vi "DM API.vi"(4 "response timeout(500)":i32=500, 6 "response":bool, 8 "error in (no error)":errorcluster, 10 "parameters":string, 11 "message":string) -> (0 "error out":errorcluster, 1 "data":variant, 2 "response":string, 3 "status":string)   [LabVIEW 2019, in "DataManagment.lvlib"]
uses:
  DataManagment.lvlib
  Intertarget communication/Command + data + response cluster.ctl
  Intertarget communication/Status + response + data cluster.ctl
  DM GV.vi
  Intertarget communication/CommandResponse communication.lvlib
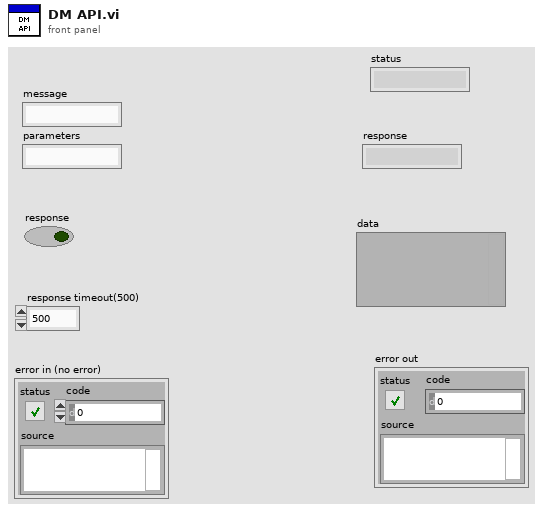
[diagram p1: front panel]
types:
  T1 = typedef "CommandResponse communication.lvlib/Status + response + data cluster.ctl" = cluster{"message":string, "response":string, "data":variant}
  T2 = typedef "CommandResponse communication.lvlib/Command + data + response cluster.ctl" = cluster{"message":string, "parameters":string, "response notifier":refnum<notifier>, "data":variant}
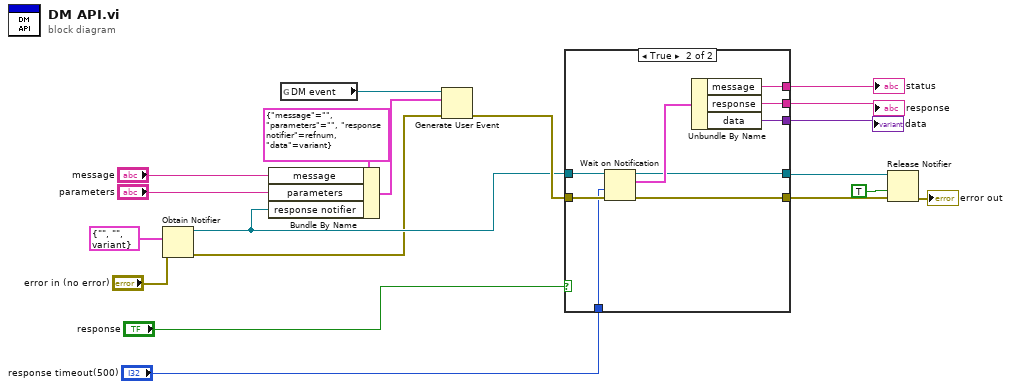
[diagram p0: block diagram]
diagram:
  n1 = Obtain Notifier(notification data type=T1 {"message"="", "response"="", "data"=variant} ("notification"), error in (no error)="error in (no error)") -> (notifier out=w15:refnum<notifier>, error out=w14:errorcluster)  [unwired: 2 in, 1 out]
  n2 = Bundle By Name(cluster=T2 {"message"="", "parameters"="", "response notifier"=refnum, "data"=variant} ("event data"), "message"="message", "parameters"="parameters", "response notifier"=w15) -> (w13:T2)
  n3 = global read "DM GV.vi" "DM event"() -> (w19:refnum<user-event>)
  n4 = Generate User Event(user event=w19, event data cluster=w13, error in=w14) -> (error out=w18:errorcluster)  [unwired: 1 in, 1 out]
  n5 = case shown="True" "response" {
    tunnel: w18 -> [w20 w30]
    tunnel: w15 -> [w21 w28]
    tunnel: [w21 w27] -> w9
    tunnel: [w20 w26] -> w7
    tunnel: [_ w25] -> w5
    tunnel: [_ w24] -> w4
    tunnel: "response timeout(500)" -> [_ w23]
    tunnel: [_ w22] -> w1
    frame False {
    }
    frame True {
      n6 = Wait on Notification(notifier=w28, timeout in ms (-1)=w23, error in (no error)=w30) -> (notifier out=w27:refnum<notifier>, notification=w29:T1, error out=w26:errorcluster)  [unwired: 1 in, 1 out]
      n7 = Unbundle By Name(w29) -> ("message"=w25:string, "response"=w24:string, "data"=w22:variant)
    }
  }
  "status" <- w5
  "response" <- w4
  "data" <- w1
  n8 = Release Notifier(notifier=w9, force destroy? (F)=TRUE, error in (no error)=w7) -> (error out=→"error out":errorcluster)  [unwired: 2 out]
